vi "MessageBall.vi"(11 "ball":T1) -> (1 "Array":u8[](array[numeric]))   [LabVIEW 2023]
uses:
  Vision_class/Old vision/SSL Detection Frame Simple Estimator Cameras VelCmd Folder/Core/AI Ball.ctl
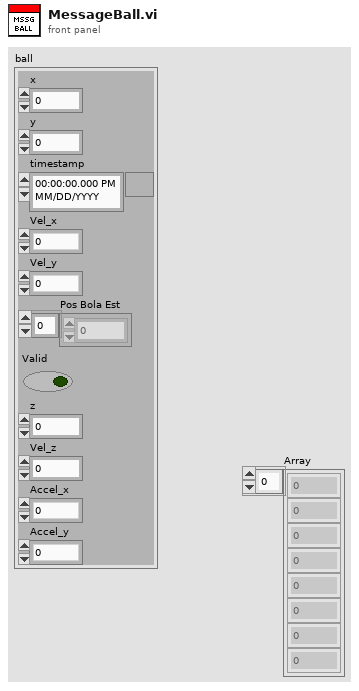
[diagram p1: front panel]
types:
  T1 = typedef "AI Ball.ctl" = cluster{"x":dbl, "y":dbl, "timestamp":timestamp, "Vel_x":dbl, "Vel_y":dbl, "Pos Bola Est":dbl[], "Valid":bool, "z":dbl, "Vel_z":dbl, "Accel_x":dbl, "Accel_y":dbl}
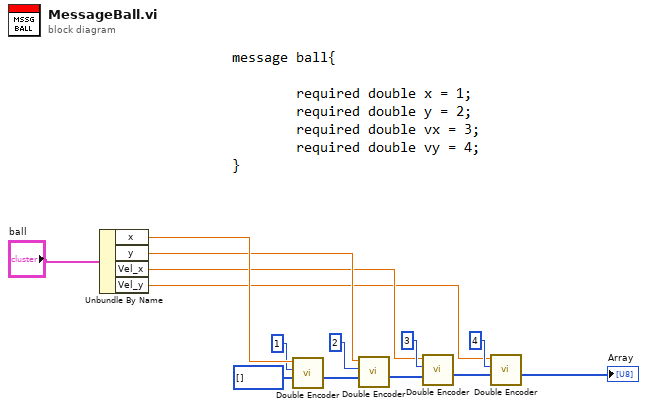
[diagram p0: block diagram]
diagram:
  n1 = Unbundle By Name("ball") -> ("x"=w14:dbl, "y"=w6:dbl, "Vel_x"=w5:dbl, "Vel_y"=w4:dbl)
  n2 = call "Double Encoder.vi"("Array In"=u8[] [], "Key"=u32 1, "Value"=w14) -> ("Array"=w11:u8[])  [unwired: 8 in]
  n3 = call "Double Encoder.vi"("Array In"=w11, "Key"=u32 2, "Value"=w6) -> ("Array"=w9:u8[])  [unwired: 8 in]
  n4 = call "Double Encoder.vi"("Array In"=w9, "Key"=u32 3, "Value"=w5) -> ("Array"=w7:u8[])  [unwired: 8 in]
  n5 = call "Double Encoder.vi"("Array In"=w7, "Key"=u32 4, "Value"=w4) -> ("Array"=→"Array":u8[])  [unwired: 8 in]
